vi "Get Controls Value and Type by Names.vi"(8 "错误输入（无错误）":errorcluster, 10 "Controls Names":string[](array[string]), 11 "VI Ref":refnum<vi>) -> (0 "错误输出":errorcluster, 2 "Enum Types":T1[](array[typedef]), 3 "Controls Value":variant[](array[variant]))   [LabVIEW 2012, in "VIRef.lvlib"]
uses:
  VIRef.lvlib
  <vilib>/Utility/VariantDataType/Type.ctl
  <vilib>/Utility/VariantDataType/VariantType.lvlib
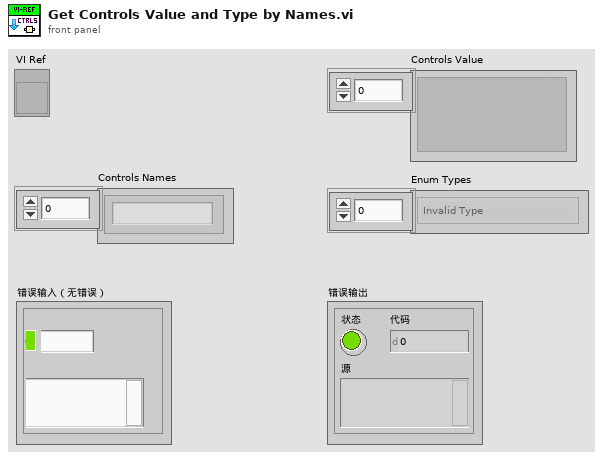
[diagram p1: front panel]
types:
  T1 = typedef "VariantType.lvlib/Type.ctl" = enum8{"Invalid Type", "Void", "I8", "I16", "I32", "I64", "U8", "U16", "U32", "U64", "Single Float", "Double Float", "Extended Float", "Single Complex", "Double Complex", "Extended Complex", "Enum U8", "Enum U16", "Enum U32", "Enum U64", "Single Float With Unit", "Double Float With Unit", "Extended Float With Unit", "Single Complex with Unit", "Double Complex with Unit", "Extended Complex with Unit", "Boolean", "String", "Path", "Picture", "Tag", "Array", "Cluster", "Variant", "LV Variant", "Waveform", "Timestamp", "Digital Waveform", "Digital Data", "ExpressData", "Refnum", "External Data", "VI", "Poly VI", "LabVIEW Class Instance", "Fixed Point"}
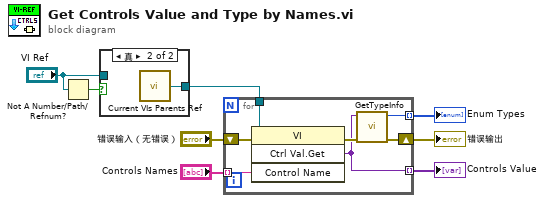
[diagram p0: block diagram]
diagram:
  n1 = Not A Number/Path/Refnum?(number/path/refnum="VI Ref") -> (NaN/Path/Refnum?=w8:bool)
  n2 = case shown="真" w8 {
    tunnel: [w9 w10] -> w6
    tunnel: "VI Ref" -> [w9 _]
    frame False {
    }
    frame True {
      n3 = call "Current VIs Parents Ref.vi"() -> ("Calling VI's Reference"=w10:refnum<vi>)  [unwired: 2 in]
    }
  }
  n4 = for {
    tunnel: w6 -> [w17]
    shift-right: [w14] -> w4
    shift-left: "错误输入（无错误）" -> [w15]
    tunnel: [w13] -> w3 mode=indexing
    tunnel: [w12] -> w2 mode=indexing
    tunnel: "Controls Names" -> [w11] mode=indexing
    n5 = invoke class="VI" method="Ctrl Val.Get"(reference=w17, error in=w15, "Control Name"=w11) -> (error out=w16:errorcluster, "Get Control Value Variant"=w12:variant)  [unwired: 1 in, 2 out]
    n6 = call <vilib>:"GetTypeInfo.vi"("error in (no error)"=w16, "Variant"=w12) -> ("error out"=w14:errorcluster, "Type Enum"=w13:T1)  [unwired: 5 in, 3 out]
  }
  "错误输出" <- w4
  "Controls Value" <- w2
  "Enum Types" <- w3
